vi "ConfigDevice.vi"(8 "error in (no error)":errorcluster, 11 "ChromaPowerSupply in":refnum<class "ChromaPowerSupply.lvclass">) -> (0 "error out":errorcluster, 3 "ChromaPowerSupply out":refnum<class "ChromaPowerSupply.lvclass">)   [LabVIEW 2018, in "AcPwrPlugins.lvlib" / "ChromaPowerSupply.lvclass"]
doc: "This VI configures all the properties set by the user through the INI file or the Properties Dialog box."
uses:
  ChromaPowerSupply.lvclass
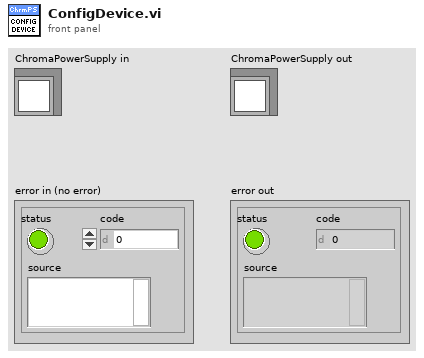
[diagram p1: front panel]
types:
  T1 = typedef "AcPwrPlugins.lvlib/ChromaPowerSupply.lvclass/Device(s)Settings.ctl" = cluster{"Phases":cluster{"Handle":string, "Instrument Options":string, "id query (T)":bool, "reset device (T)":bool, "Timing":cluster{"TimingOn":enum16{""}, "Hours":u32, "Minutes":u32, "Seconds":dbl, "CutoffVoltage":dbl}, "Connected":bool, "Output Mode":enum16{"Voltage (DC)", "Current (DC)"}, "Voltage":dbl, "Current":dbl, "Voltage Limit":dbl, "Current Limit":dbl, "Power Protect":dbl, "Current Protect":dbl, "Voltage Protect":dbl}[], "MeasName":string}
  T2 = cluster{"Handle":string, "Instrument Options":string, "id query (T)":bool, "reset device (T)":bool, "Timing":cluster{"TimingOn":enum16{""}, "Hours":u32, "Minutes":u32, "Seconds":dbl, "CutoffVoltage":dbl}, "Connected":bool, "Output Mode":enum16{"Voltage (DC)", "Current (DC)"}, "Voltage":dbl, "Current":dbl, "Voltage Limit":dbl, "Current Limit":dbl, "Power Protect":dbl, "Current Protect":dbl, "Voltage Protect":dbl}[]
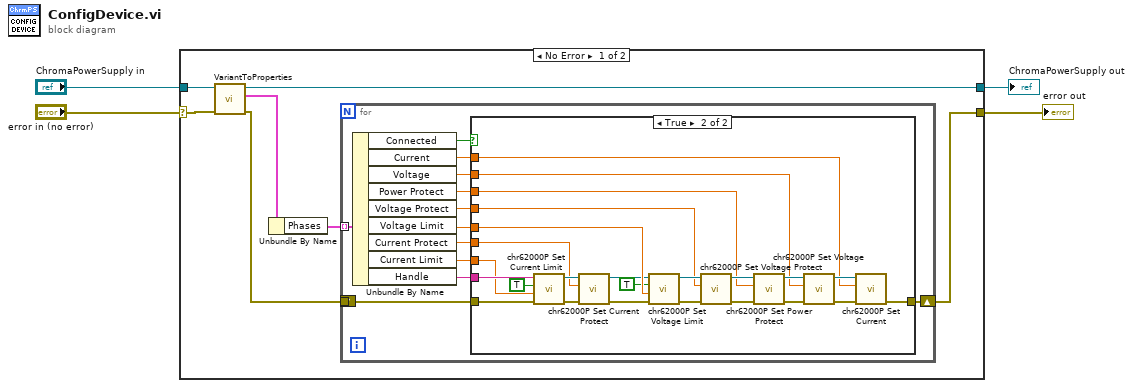
[diagram p0: block diagram]
diagram:
  n1 = case shown="No Error" "error in (no error)" {
    selector: "error in (no error)" -> [w10 w49]
    tunnel: "ChromaPowerSupply in" -> [w11 w50]
    tunnel: [w9 w50] -> w2
    tunnel: [w5 w49] -> w1
    frame No Error {
      n2 = call-dynamic "VariantToProperties.vi"("error in (no error)"=w10, "ChromaPowerSupply in"=w11) -> ("error out"=w6:errorcluster, "Device Settings"=w8:T1, "ChromaPowerSupply out"=w9:refnum<class "ChromaPowerSupply.lvclass">)  [unwired: 5 in, 2 out]
      n3 = Unbundle By Name(w8) -> ("Phases"=w7:T2)
      n4 = for {
        tunnel: w7 -> [w23] mode=indexing
        tunnel: w6 -> [w21]
        shift-right: [w18] -> w5
        shift-left: _ -> [_]
        n5 = Unbundle By Name(w23) -> ("Connected"=w14:bool, "Current"=w12:dbl, "Voltage"=w13:dbl, "Power Protect"=w15:dbl, "Voltage Protect"=w17:dbl, "Voltage Limit"=w19:dbl, "Current Protect"=w16:dbl, "Current Limit"=w20:dbl, "Handle"=w22:string)
        n6 = case shown="True" w14 {
          tunnel: w22 -> [_ w48]
          tunnel: w21 -> [w24 w47]
          tunnel: w20 -> [_ w39]
          tunnel: w19 -> [_ w46]
          tunnel: [w24 w27] -> w18
          tunnel: w17 -> [_ w35]
          tunnel: w16 -> [_ w38]
          tunnel: w15 -> [_ w32]
          tunnel: w13 -> [_ w26]
          tunnel: w12 -> [_ w25]
          frame False {
          }
          frame True {
            n7 = call <instrlib>:"chr62000P Set Current Limit.vi"("error in (no error)"=w47, "Current Limit (0.0)"=w39, "High/Low (Low)"=TRUE, "instrument handle"=w48) -> ("error out"=w42:errorcluster, "instrument handle out"=w43:refnum<k15>)  [unwired: 6 in]
            n8 = call <instrlib>:"chr62000P Set Current Protect.vi"("error in (no error)"=w42, "Current Protect (63.0)"=w38, "instrument handle"=w43) -> ("error out"=w40:errorcluster, "instrument handle out"=w41:refnum<k15>)  [unwired: 7 in]
            n9 = call <instrlib>:"chr62000P Set Voltage Limit.vi"("error in (no error)"=w40, "Voltage Limit (0.0)"=w46, "High/Low (Low)"=TRUE, "instrument handle"=w41) -> ("error out"=w37:errorcluster, "instrument handle out"=w36:refnum<k15>)  [unwired: 6 in]
            n10 = call <instrlib>:"chr62000P Set Voltage Protect.vi"("error in (no error)"=w37, "Voltage Protect (88.0)"=w35, "instrument handle"=w36) -> ("error out"=w34:errorcluster, "instrument handle out"=w33:refnum<k15>)  [unwired: 7 in]
            n11 = call <instrlib>:"chr62000P Set Power Protect.vi"("error in (no error)"=w34, "Power Protect (1260.0)"=w32, "instrument handle"=w33) -> ("error out"=w30:errorcluster, "instrument handle out"=w31:refnum<k15>)  [unwired: 7 in]
            n12 = call <instrlib>:"chr62000P Set Voltage.vi"("error in (no error)"=w30, "Voltage (0.00)"=w26, "instrument handle"=w31) -> ("error out"=w28:errorcluster, "instrument handle out"=w29:refnum<k15>)  [unwired: 7 in]
            n13 = call <instrlib>:"chr62000P Set Current.vi"("error in (no error)"=w28, "Current (0.00)"=w25, "instrument handle"=w29) -> ("error out"=w27:errorcluster)  [unwired: 7 in, 1 out]
          }
        }
      }
    }
    frame Error {
    }
  }
  "error out" <- w1
  "ChromaPowerSupply out" <- w2
